vi "XY Graph Special Event Handler Core.vi"(8 "error in (no error)":errorcluster, 11 "XY Graph Event":T1) -> (0 "error out":errorcluster, 1 "Data":variant, 2 "Message":string, 3 "Menu Item Tag (dup)":string, 5 "Top Menu":string)   [LabVIEW 2019, in "XY Graph Add-Ons.lvlib"]
uses:
  XY Graph Add-Ons.lvlib
  XY Graph Event.ctl
  <vilib>/Utility/miscctls.llb/LVPoint32TypeDef.ctl
  Fits/Fit Plot Request Information.ctl
  <vilib>/Utility/miscctls.llb/LVPointDoubleTypeDef.ctl
  Fits/Fit Models.ctl
  XY Graph Mouse Click Event Data.ctl
  XY Graph Refnum.ctl
  Plot Editor/Plot Editor.lvlib
  Histograms/Histogram Window.lvlib
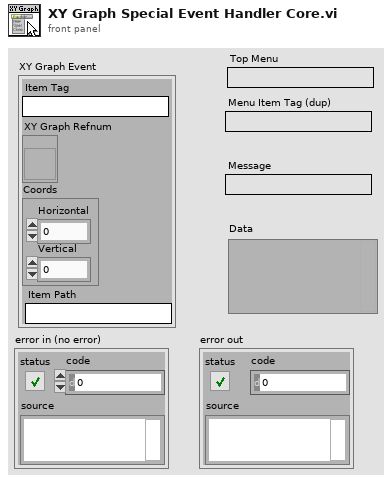
[diagram p1: front panel]
types:
  T1 = typedef "XY Graph Add-Ons.lvlib/XY Graph Event.ctl" = cluster{"Item Tag":string, "XY Graph Refnum":refnum<vi>, "Coords":T2, "Item Path":string}
  T2 = typedef "LVPoint32TypeDef.ctl" = cluster{"Horizontal":i32, "Vertical":i32}
  T3 = typedef "Fit Plot Request Information.ctl" = cluster{"XY Graph Ref":refnum<vi>, "Mouse Coordinates":T4, "Fit Model":T5, "Plot Index":i32}
  T4 = typedef "LVPointDoubleTypeDef.ctl" = cluster{"X":dbl, "Y":dbl}
  T5 = typedef "Fit Models.ctl" = enum16{"Select a Fit Model...", "           Single Peak", "Gaussian", "Asymmetric Gaussian", "Lorentzian", "Asymmetric Lorentzian", "Gaussian/Lorentzian", "Lorentzian/Gaussian", "           Double Peak", "Two Gaussians", "Two Asymmetric Gaussians", "Two H-Connected Gaussians", "Two T-Connected Gaussians", "Two H-Connected Asymmetric Gaussians", "Two T-Connected Asymmetric Gaussians", "           Triple Peak", "Three Gaussians", "Three Asymmetric Gaussians", "              Decays", "1-Exponential", "IRF*PSED", "2-Exponentials", "               ACF", "2D Gaussian ACF", "2D Gaussian + Blinking ACF", "2D Gaussian + Flow ACF", "3D Gaussian ACF", "3D Gaussian + Blinking ACF", "             Multiplot", "2D Gaussian ACF & 2D Gaussian + Flow ACF"}
  T6 = typedef "XY Graph Add-Ons.lvlib/XY Graph Mouse Click Event Data.ctl" = cluster{"Multiplot XY Graph":T7, "Mouse Coordinates":T2}
  T7 = typedef "XY Graph Add-Ons.lvlib/XY Graph Refnum.ctl" = refnum<vi>
  T8 = typedef "Plot Style 3.ctl" = cluster{"Plot Style":enum16{"unchanged", "Line", "Symbol", "Line + Symbol", "Histogram", "Histogram + Symbol"}, "Histogram Type":enum16{"unchanged", "Left Bound", "Center", "Right Bound"}, "Line Tickness":enum16{"unchanged", "Thin", "1 pixel", "2 pixel", "3 pixel", "4 pixel", "5 pixel"}, "Line Style":enum16{"unchanged", "Plain", "Long Dash", "Short Dash", "Long-Short Dash", "Long-Short-Short Dash"}, "Point Style":enum16{"unchanged", "None", "Empty Circle", "Filled Circle", "Thick Circle", "Dotted Circle", "Empty Square", "Filled Square", "Thick Square", "Dotted Square", "Small Filled Square", "Dot", "Cross", "Tiny Cross", "Large X", "Small x", "Diamond", "Small Empty Square"}, "Line Color":u32, "Point Color":u32, "Anti-aliased":bool, "Line Color Chooser":enum16{"unchanged", "Color Box", "Color List"}, "Point Color Chooser":enum16{"unchanged", "Color Box", "Color List"}, "Line Color List":string, "Point Color List":string}
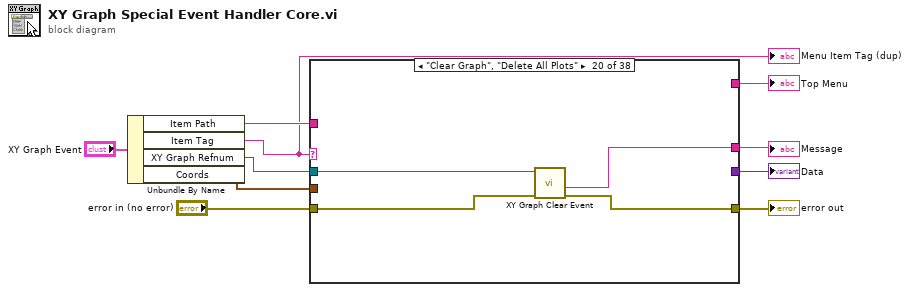
[diagram p0: block diagram]
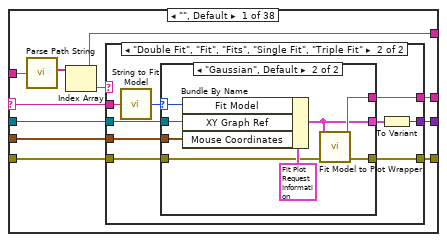
[diagram p2: hidden frame]
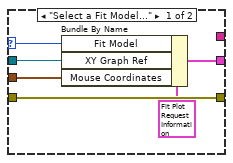
[diagram p4: hidden frame]
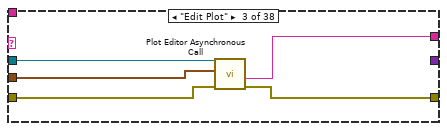
[diagram p6: hidden frame]
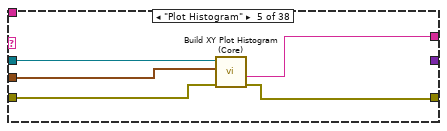
[diagram p8: hidden frame]
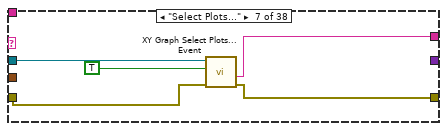
[diagram p10: hidden frame]
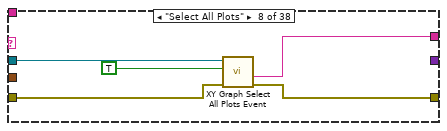
[diagram p11: hidden frame]
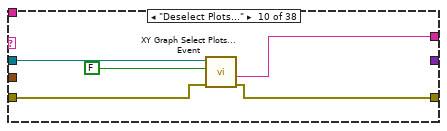
[diagram p13: hidden frame]
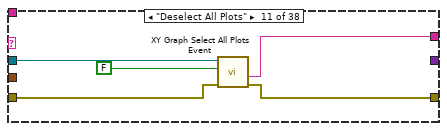
[diagram p14: hidden frame]
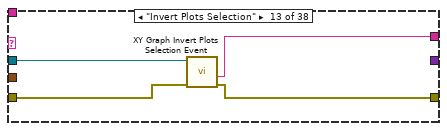
[diagram p16: hidden frame]
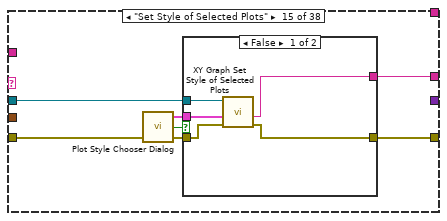
[diagram p18: hidden frame]
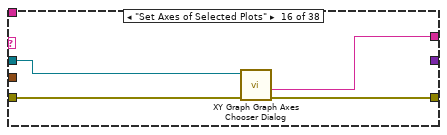
[diagram p20: hidden frame]
diagram:
  n1 = Unbundle By Name("XY Graph Event") -> ("Item Path"=w5:string, "Item Tag"=w4:string, "XY Graph Refnum"=w3:refnum<vi>, "Coords"=w2:T2)
  "Menu Item Tag (dup)" <- w4
  n2 = case shown="\"Clear Graph\", \"Delete All Plots\"" w4 {
    selector: w4 -> [w18 _ _ _ _ _ _ _ _ _ _ _ _ _ _ _ _ _ _ _ _ _ _ _ _ _ _ _ _ _ _ _ _ _ _ _ _ _]
    tunnel: w3 -> [w20 _ w50 _ w56 _ w62 w67 _ w73 w78 _ w83 _ w88 w99 _ w109 w115 w119 _ w123 w129 w134 _ w143 _ w150 _ w157 w162 _ w170 w177 w184 _ w189 w193]
    tunnel: w2 -> [w19 _ w49 _ w55 _ _ _ _ _ _ _ _ _ _ _ _ w108 _ _ _ w124 _ _ _ _ _ w149 _ _ _ _ w169 w176 w183 _ _ _]
    tunnel: "error in (no error)" -> [w15 w45 w48 w51 w54 w57 w61 w65 w68 w72 w76 w79 w82 w84 w87 w101 w102 w107 w114 w118 w120 w125 w130 w135 w136 w142 w144 w147 w152 w154 w159 w163 w167 w174 w181 w185 w188 w192]
    tunnel: [w14 w45 w47 w51 w53 w57 w59 w63 w68 w70 w74 w79 w81 w84 w86 w100 w102 w105 w113 w117 w120 w122 w128 w133 w136 w141 w144 w146 w152 w155 w160 w163 w166 w173 w180 w185 w187 w191] -> w9
    tunnel: [w13 _ w46 _ w52 _ w58 w64 _ w69 w75 _ w80 _ w85 w98 _ w106 w112 w116 _ w121 w126 w131 _ w140 _ w145 _ w153 w158 _ w165 w172 w179 _ w186 w190] -> w10
    tunnel: w5 -> [w17 _ _ _ _ _ _ _ _ _ _ _ _ _ _ _ _ _ _ _ _ _ _ _ _ _ _ _ _ _ _ _ _ _ _ _ _ _]
    tunnel: [w12 _ _ _ _ _ _ _ _ _ _ _ _ _ _ _ _ w103 w110 _ _ _ _ _ _ w139 _ _ _ _ _ _ _ _ _ _ _ _] -> w7
    tunnel: [w11 _ _ _ _ _ _ _ _ _ _ _ _ _ _ _ _ _ _ _ _ _ _ _ _ _ _ _ _ _ _ _ _ _ _ _ _ _] -> w1
    frame "", Default {
      (unwired) T3 {"XY Graph Ref"=refnum, "Mouse Coordinates"={"X"=0.0, "Y"=0.0}, "Fit Model"=enum."Select a Fit Model...", "Plot Index"=-1} ("output cluster")
      n3 = call "Parse Path String.vi"("Path in"=w17) -> ("Folder Hierarchy"=w16:string[])  [unwired: 4 in, 1 out]
      n4 = Index Array(array=w16) -> (element=w11:string)  [unwired: 1 in]
      n5 = case shown="\"Double Fit\", \"Fit\", \"Fits\", \"Single Fit\", \"Triple Fit\"" w11 {
        tunnel: w20 -> [_ w30]
        tunnel: w19 -> [_ w29]
        tunnel: w18 -> [_ w28]
        tunnel: w15 -> [w21 w26]
        tunnel: [w21 w25] -> w14
        tunnel: [_ w24] -> w13
        tunnel: [_ w22] -> w12
        frame "", Default {
        }
        frame "Double Fit", "Fit", "Fits", "Single Fit", "Triple Fit" {
          n6 = call "String to Fit Model.vi"("String"=w28) -> ("Fit Model"=w27:T5)  [unwired: 8 in]
          n7 = case shown="\"Gaussian\", Default" w27 {
            selector: w27 -> [w35 w41]
            tunnel: w30 -> [w34 w42]
            tunnel: w29 -> [w33 w43]
            tunnel: w26 -> [w36 w40]
            tunnel: [w36 w39] -> w25
            tunnel: [_ w38] -> w24
            tunnel: [w31 w37] -> w23
            frame "Select a Fit Model..." {
              n8 = Bundle By Name(cluster=T3 {"XY Graph Ref"=refnum, "Mouse Coordinates"={"X"=0.0, "Y"=0.0}, "Fit Model"=enum."Select a Fit Model...", "Plot Index"=0} ("Fit Plot Info"), "Fit Model"=w35, "XY Graph Ref"=w34, "Mouse Coordinates"=w33) -> (w31:T3)
            }
            frame "Gaussian", Default {
              n9 = Bundle By Name(cluster=T3 {"XY Graph Ref"=refnum, "Mouse Coordinates"={"X"=0.0, "Y"=0.0}, "Fit Model"=enum."Select a Fit Model...", "Plot Index"=-1} ("output cluster"), "Fit Model"=w41, "XY Graph Ref"=w42, "Mouse Coordinates"=w43) -> (w37:T3)
              n10 = call "Fit Model to Plot Wrapper.vi"("error in (no error)"=w40, "Fit Plot Info"=w37) -> ("error out"=w39:errorcluster, "Fit Result String"=w38:string)  [unwired: 8 in]
            }
          }
          n11 = To Variant(anything=w23) -> (Variant=w22:variant)
        }
      }
    }
    frame "---------" {
    }
    frame "Edit Plot" {
      n12 = call "Plot Editor Asynchronous Call.vi"("error in (no error)"=w48, "Coords"=w49, "XYGraph in"=w50) -> ("Error Out"=w47:errorcluster, "Message"=w46:string)  [unwired: 5 in, 2 out]
    }
    frame "-------------" {
    }
    frame "Plot Histogram" {
      n13 = call "Build XY Plot Histogram (Core).vi"("error in (no error)"=w54, "Mouse Click Coords"=w55, "XYGraph in"=w56) -> ("error out"=w53:errorcluster, "Message"=w52:string)  [unwired: 6 in, 1 out]
    }
    frame "----------------" {
    }
    frame "Select Plots..." {
      n14 = call "XY Graph Select Plots... Event.vi"("Error In"=w61, "Select (T)/Deselect"=TRUE, "XYGraph Ref"=w62) -> ("Error Out"=w59:errorcluster, "Message"=w58:string)  [unwired: 4 in, 3 out]
    }
    frame "Select All Plots" {
      n15 = call "XY Graph Select All Plots Event.vi"("Error In"=w65, "Select (T)/Deselect"=TRUE, "XYGraph Ref"=w67) -> ("Error Out"=w63:errorcluster, "Message"=w64:string)  [unwired: 5 in, 2 out]
    }
    frame "----------------------" {
    }
    frame "Deselect Plots..." {
      n16 = call "XY Graph Select Plots... Event.vi"("Error In"=w72, "Select (T)/Deselect"=FALSE, "XYGraph Ref"=w73) -> ("Error Out"=w70:errorcluster, "Message"=w69:string)  [unwired: 4 in, 3 out]
    }
    frame "Deselect All Plots" {
      n17 = call "XY Graph Select All Plots Event.vi"("Error In"=w76, "Select (T)/Deselect"=FALSE, "XYGraph Ref"=w78) -> ("Error Out"=w74:errorcluster, "Message"=w75:string)  [unwired: 5 in, 2 out]
    }
    frame "-----------------------" {
    }
    frame "Invert Plots Selection" {
      n18 = call "XY Graph Invert Plots Selection Event.vi"("Error In"=w82, "XYGraph Ref"=w83) -> ("Error Out"=w81:errorcluster, "Message"=w80:string)  [unwired: 6 in, 2 out]
    }
    frame "---------------" {
    }
    frame "Set Style of Selected Plots" {
      n19 = call "Plot Style Chooser Dialog.vi"("Error In"=w87) -> ("Plot Style out"=w91:T8, "Cancelled?"=w90:bool, "Error Out"=w89:errorcluster)  [unwired: 6 in]
      n20 = case shown="False" w90 {
        tunnel: w88 -> [w96 _]
        tunnel: w91 -> [w95 _]
        tunnel: w89 -> [w94 w97]
        tunnel: [w93 w97] -> w86
        tunnel: [w92 _] -> w85
        frame False {
          n21 = call "XY Graph Set Style of Selected Plots.vi"("Error In"=w94, "Plot Style"=w95, "XYGraph Ref"=w96) -> ("Error Out"=w93:errorcluster, "Message"=w92:string)  [unwired: 5 in, 2 out]
        }
        frame True {
        }
      }
    }
    frame "Set Axes of Selected Plots" {
      n22 = call "XY Graph Graph Axes Chooser Dialog.vi"("Error In"=w101, "XYGraph Ref"=w99) -> ("Error Out"=w100:errorcluster, "Message"=w98:string)  [unwired: 6 in, 2 out]
    }
    frame "-----------------" {
    }
    frame "Delete Plot" {
      n23 = call "XY Graph Delete Plot Event.vi"("Error In"=w107, "Mouse Click Coordinates"=w108, "XYGraph Ref"=w109) -> ("Error Out"=w105:errorcluster, "Message"=w106:string, "Deleted Plot Index"=w104:i32)  [unwired: 4 in, 2 out]
      n24 = To Variant(anything=w104) -> (Variant=w103:variant)
    }
    frame "Delete Selected Plots" {
      n25 = call "XY Graph Delete Selected Plots Event.vi"("Error In"=w114, "XYGraph Ref"=w115) -> ("Error Out"=w113:errorcluster, "Message"=w112:string, "Deleted Plot Indices"=w111:i32[])  [unwired: 5 in, 2 out]
      n26 = To Variant(anything=w111) -> (Variant=w110:variant)
    }
    frame "Clear Graph", "Delete All Plots" {
      n27 = call "XY Graph Clear Event.vi"("Error In"=w118, "XYGraph Ref"=w119) -> ("Error Out"=w117:errorcluster, "Message"=w116:string)  [unwired: 7 in, 1 out]
    }
    frame "------------------" {
    }
    frame "Save Plot" {
      n28 = call "XY Graph Save Plot Event.vi"("Error In"=w125, "Mouse Click Coordinates"=w124, "XYGraph Ref"=w123) -> ("Error Out"=w122:errorcluster, "Message"=w121:string)  [unwired: 3 in, 4 out]
    }
    frame "Save Selected Plots" {
      n29 = call "XY Graph Save Selected Plots Event.vi"("Error In"=w130, "Save All Plots? (T)"=FALSE, "XYGraph Ref"=w129) -> ("Error Out"=w128:errorcluster, "Message"=w126:string)  [unwired: 3 in, 4 out]
    }
    frame "Save All Plots" {
      n30 = call "XY Graph Save Selected Plots Event.vi"("Error In"=w135, "Save All Plots? (T)"=TRUE, "XYGraph Ref"=w134) -> ("Error Out"=w133:errorcluster, "Message"=w131:string)  [unwired: 3 in, 4 out]
    }
    frame "------------" {
    }
    frame "Load Plot(s)" {
      n31 = call "XY Graph Load Plot(s) Event.vi"("Error In"=w142, "XYGraph Ref"=w143) -> ("Error Out"=w141:errorcluster, "Message"=w140:string, "# Plots Added"=w138:i32[])  [unwired: 4 in, 3 out]
      n32 = Add Array Elements(numeric array=w138) -> (sum=w137:i32)
      n33 = To Variant(anything=w137) -> (Variant=w139:variant)
    }
    frame "--------------------------" {
    }
    frame "Transpose Plot" {
      n34 = Bundle(cluster=T6 {"Multiplot XY Graph"=refnum, "Mouse Coordinates"={"Horizontal"=0, "Vertical"=0}} ("Mouse Click Event Data"), "Multiplot XY Graph"=w150, "Mouse Coordinates"=w149) -> (w148:T6)
      n35 = call "XY Graph Transpose Plot Event.vi"("Error In"=w147, "Mouse Click Event Data"=w148) -> ("Error Out"=w146:errorcluster, "Message"=w145:string)  [unwired: 6 in, 2 out]
    }
    frame "--------------------" {
    }
    frame "Add Selected Plots" {
      n36 = call "XY Graph Sum Selected Plots Event.vi"("Error In"=w154, "Add All Plots? (F)"=FALSE, "XYGraph Ref"=w157) -> ("Error Out"=w155:errorcluster, "Message"=w153:string)  [unwired: 3 in, 4 out]
    }
    frame "Add All Plots" {
      n37 = call "XY Graph Sum Selected Plots Event.vi"("Error In"=w159, "Add All Plots? (F)"=TRUE, "XYGraph Ref"=w162) -> ("Error Out"=w160:errorcluster, "Message"=w158:string)  [unwired: 3 in, 4 out]
    }
    frame "---------------------" {
    }
    frame "Plot Arithmetic", "Single Plot Arithmetic", "y >> f(y) Transform" {
      n38 = Bundle(cluster=T6 {"Multiplot XY Graph"=refnum, "Mouse Coordinates"={"Horizontal"=0, "Vertical"=0}} ("Mouse Click Event Data"), "Multiplot XY Graph"=w170, "Mouse Coordinates"=w169) -> (w168:T6)
      n39 = call "XY Graph Compute Simple Plot Formula Event.vi"("Error In"=w167, "Mouse Click Event Data"=w168) -> ("Error Out"=w166:errorcluster, "Message"=w165:string)  [unwired: 5 in, 3 out]
    }
    frame "Interpolate Plot" {
      n40 = Bundle(cluster=T6 {"Multiplot XY Graph"=refnum, "Mouse Coordinates"={"Horizontal"=0, "Vertical"=0}} ("Mouse Click Event Data"), "Multiplot XY Graph"=w177, "Mouse Coordinates"=w176) -> (w175:T6)
      n41 = call "XY Graph Interpolate Plot Event.vi"("Error In"=w174, "Mouse Click Event Data"=w175) -> ("Error Out"=w173:errorcluster, "Message"=w172:string)  [unwired: 6 in, 2 out]
    }
    frame "(x, y) >> (f, g)(x, y) Transform", "Plot Transform", "Single Plot Transform" {
      n42 = Bundle(cluster=T6 {"Multiplot XY Graph"=refnum, "Mouse Coordinates"={"Horizontal"=0, "Vertical"=0}} ("Mouse Click Event Data"), "Multiplot XY Graph"=w184, "Mouse Coordinates"=w183) -> (w182:T6)
      n43 = call "XY Graph Compute Complex Plot Formula Event.vi"("Error In"=w181, "Mouse Click Event Data"=w182) -> ("Error Out"=w180:errorcluster, "Message"=w179:string)  [unwired: 5 in, 3 out]
    }
    frame "-------------------" {
    }
    frame "Grid", "Show/Hide Grid" {
      n44 = call "XY Graph Show-Hide Grid Event.vi"("Error In"=w188, "XYGraph Ref in"=w189) -> ("Error Out"=w187:errorcluster, "Message"=w186:string)  [unwired: 6 in, 2 out]
    }
    frame "Show/Hide Tool Panels", "Tool Panels" {
      n45 = call "XY Graph Show-Hide Tool Panels Event.vi"("Error In"=w192, "XYGraph in"=w193) -> ("Error Out"=w191:errorcluster, "Message"=w190:string)  [unwired: 7 in, 1 out]
    }
  }
  "Message" <- w10
  "error out" <- w9
  "Data" <- w7
  "Top Menu" <- w1
